vi "滴定曲线.vi"() -> ()   [LabVIEW 2016]
panel:
  out "ORP滴定曲线":u16[](graph)
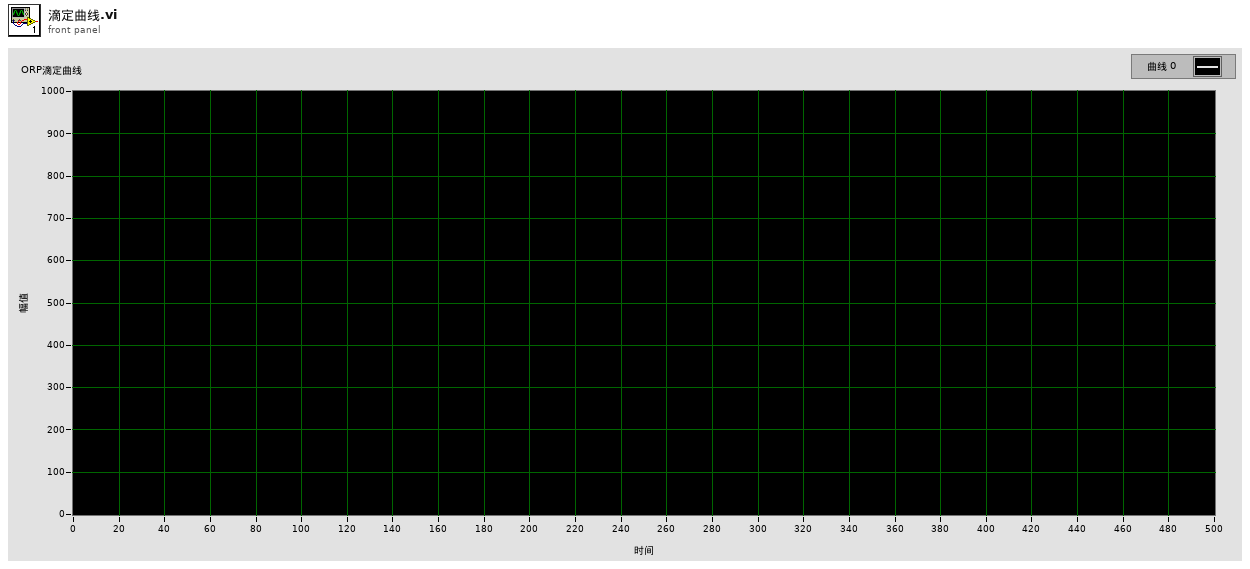
[diagram p1: front panel]
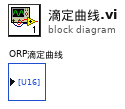
[diagram p0: block diagram]
diagram:
